vi "MainV2.vi"() -> ()   [LabVIEW 2010]
uses:
  <vilib>/Instr/_visa.llb/VISA Set IO Buffer Mask.ctl
  <vilib>/Instr/_visa.llb/VISA Flush IO Buffer Mask.ctl
  GlobalVar.vi
  <vilib>/Instr/_visa.llb/VISA Configure Serial Port (Instr).vi
panel:
  in  "Port Com":refnum<visa-resource-name>="COM7" caption="Nom de ressource VISA"
  in  "Bouton OK":bool
  in  "Data to send":dbl
  in  "Command type":u16(ring) items=["PRET"=53, "COEF_COURANT_2_INF"=36, "COEF_COURANT_2_CON"=164, "COEF_COURANT_1_INF"=35, "COEF_COURANT_1_CON"=163, "COEF_HYSTERISIS_SECURITE_INF"=34, "POURCENT_SECURITE_MOTEUR_INF"=33, "VITESSE_TROTTOIR_MAX_INF"=32, "DEMARRAGE_DELAI_EQUILIBRE_INF"=31, "DEMARRAGE_TOL_GUIDON_INF"=30, "DEMARRAGE_TOL_ANGLE_INF"=29, "LIMITE_DISTANCE_UTILISATEUR_INF"=28, "GUIDONMAX_INF"=27, "ACCELERATION_COEF_FILTRE_INF"=26, "COEF_KALMAN_INF"=25, "PRINC_DIR_INF"=24, "PRINC_PID_D_INF"=23, "PRINC_PID_K_INF"=22, "COEF_HYSTERISIS_SECURITE_CON"=162, "POURCENT_SECURITE_MOTEUR_CON"=161, "VITESSE_TROTTOIR_MAX_CON"=160, "DEMARRAGE_DELAI_EQUILIBRE_CON"=159, "DEMARRAGE_TOL_GUIDON_CON"=158, "DEMARRAGE_TOL_ANGLE_CON"=157, "LIMITE_DISTANCE_UTILISATEUR_CON"=156, "GUIDONMAX_CON"=155, "ACCELERATION_COEF_FILTRE_CON"=154, "COEF_KALMAN_CON"=153, "PRINC_DIR_CON"=152, "PRINC_PID_D_CON"=151, "PRINC_PID_K_CON"=150, "ENREGISTER_DEMARRAGE"=149, "CHARGER_DEMARRAGE"=148, "ENREGISTRER_ASSERVISSEMENT"=147, "CHARGER_ASSERVISSEMENT"=146, "ENREGISTRER_VITESSE"=145, "CHARGER_VITESSE"=144, "DEMANDE_COEFFICIENTS"=137, "VERBOSE_INF"=8, "VERBOSE_CON"=136, "ETAT"=1, "STOP"=131, "DEPART"=130, "TEST_COM"=129]
  out "LongToSend":u8
  out "TypeToSend":u8
  out "DataToSend":u8[](array[numeric])
  out "Frequency":dbl
  out "Enum":T1(ring)
  out "error":errorcluster
  out "error Connexion":errorcluster
  out "Stop main loop":bool
  in  "stop":bool
  in  "Tab Control":T2(tab)
  out "Reception":string
  in  "Comm_BaudRate":u32=9600 caption="Baud rate"
  in  "Comm_PortComm":refnum<visa-resource-name>="COM7" caption="Communication Port"
  in  "timeout (10sec)":u32=10000
  in  "Con_RefreshIntensity":bool caption="Bouton OK 12"
  in  "Con_RefreshRightTorque":bool caption="Bouton OK 12"
  out "Con_XYIntensity":cluster{"Y":dbl[], "Y":dbl[]}[](graph) caption="Intensity"
  out "Con_XYRightTorque":cluster{"Y":dbl[], "Y":dbl[]}[](graph) caption="Motor right Torque"
  in  "Con_RefreshLeftTorque":bool caption="Bouton OK 12"
  out "Con_XYLeftTorque":cluster{"Y":dbl[], "Y":dbl[]}[](graph) caption="Motor left Torque"
  out "Con_IntensityMax":bool caption="Max Intensity"
  out "Con_Intensity":string[][](array[string]) caption="Intensity (A)"
  out "Con_MotorRightTorque":string[][](array[string]) caption="Motor right Torque (N.m)"
  out "Con_MotorLeftTorque":string[][](array[string]) caption="Motor left Torque (N.m)"
  in  "Ana_RefreshBattery":bool caption="Bouton OK 12"
  out "Ana_XYBattery":cluster{"Y":dbl[], "Y":dbl[]}[](graph) caption="Motor left Torque"
  in  "Ana_RefreshHandlebar":bool caption="Bouton OK 12"
  out "Ana_XYHandlebar":cluster{"Y":dbl[], "Y":dbl[]}[](graph) caption="Motor left Torque"
  out "Ana_Battery":string[][](array[string]) caption="Battery"
  out "Ana_Handlebar":string[][](array[string]) caption="Handlebar"
  in  "Inc_RefreshAcceleration":bool caption="Bouton OK 12"
  out "Inc_XYAcceleration":cluster{"Y":dbl[], "Y":dbl[]}[](graph) caption="Motor left Torque"
  in  "Inc_RefreshVelocityRightMotor":bool caption="Bouton OK 12"
  out "Inc_XYVelocityRightMotor":cluster{"Y":dbl[], "Y":dbl[]}[](graph) caption="Motor left Torque"
  in  "Inc_RefreshVelocityLeftMotor":bool caption="Bouton OK 12"
  out "Inc_XYVelocityLeftMotor":cluster{"Y":dbl[], "Y":dbl[]}[](graph) caption="Motor left Torque"
  out "Inc_Acceleration":string[][](array[string]) caption="Acceleration"
  out "Inc_VelocityRightMotor":string[][](array[string]) caption="Velocity Right motor"
  out "Inc_VelocityLeftMotor":string[][](array[string]) caption="Velocity left motor"
  out "Other_AngularVelocity":string[][](array[string]) caption="Angular velocity"
  out "Other_AngleOUT":string[][](array[string]) caption="Angle Out of range"
  out "Other_SpeedSaturation":string[][](array[string]) caption="Speed saturation"
  out "Other_Distance":string[][](array[string]) caption="Distance"
  out "Other_Angle":string[][](array[string]) caption="Angle"
  in  "Analyse_Time":dbl caption="Time"
  in  "Analyse_Step":dbl caption="Step"
  in  "Analyse_LeftOrRight":bool caption="Booléen"
  out "Analyse_XYTorque":cluster{"Y":dbl[], "Y":dbl[]}[](graph) caption="Motor Torque command"
  out "Analyse_MotorTorque":string[][](array[string]) caption="Motor  Torque (N.m)"
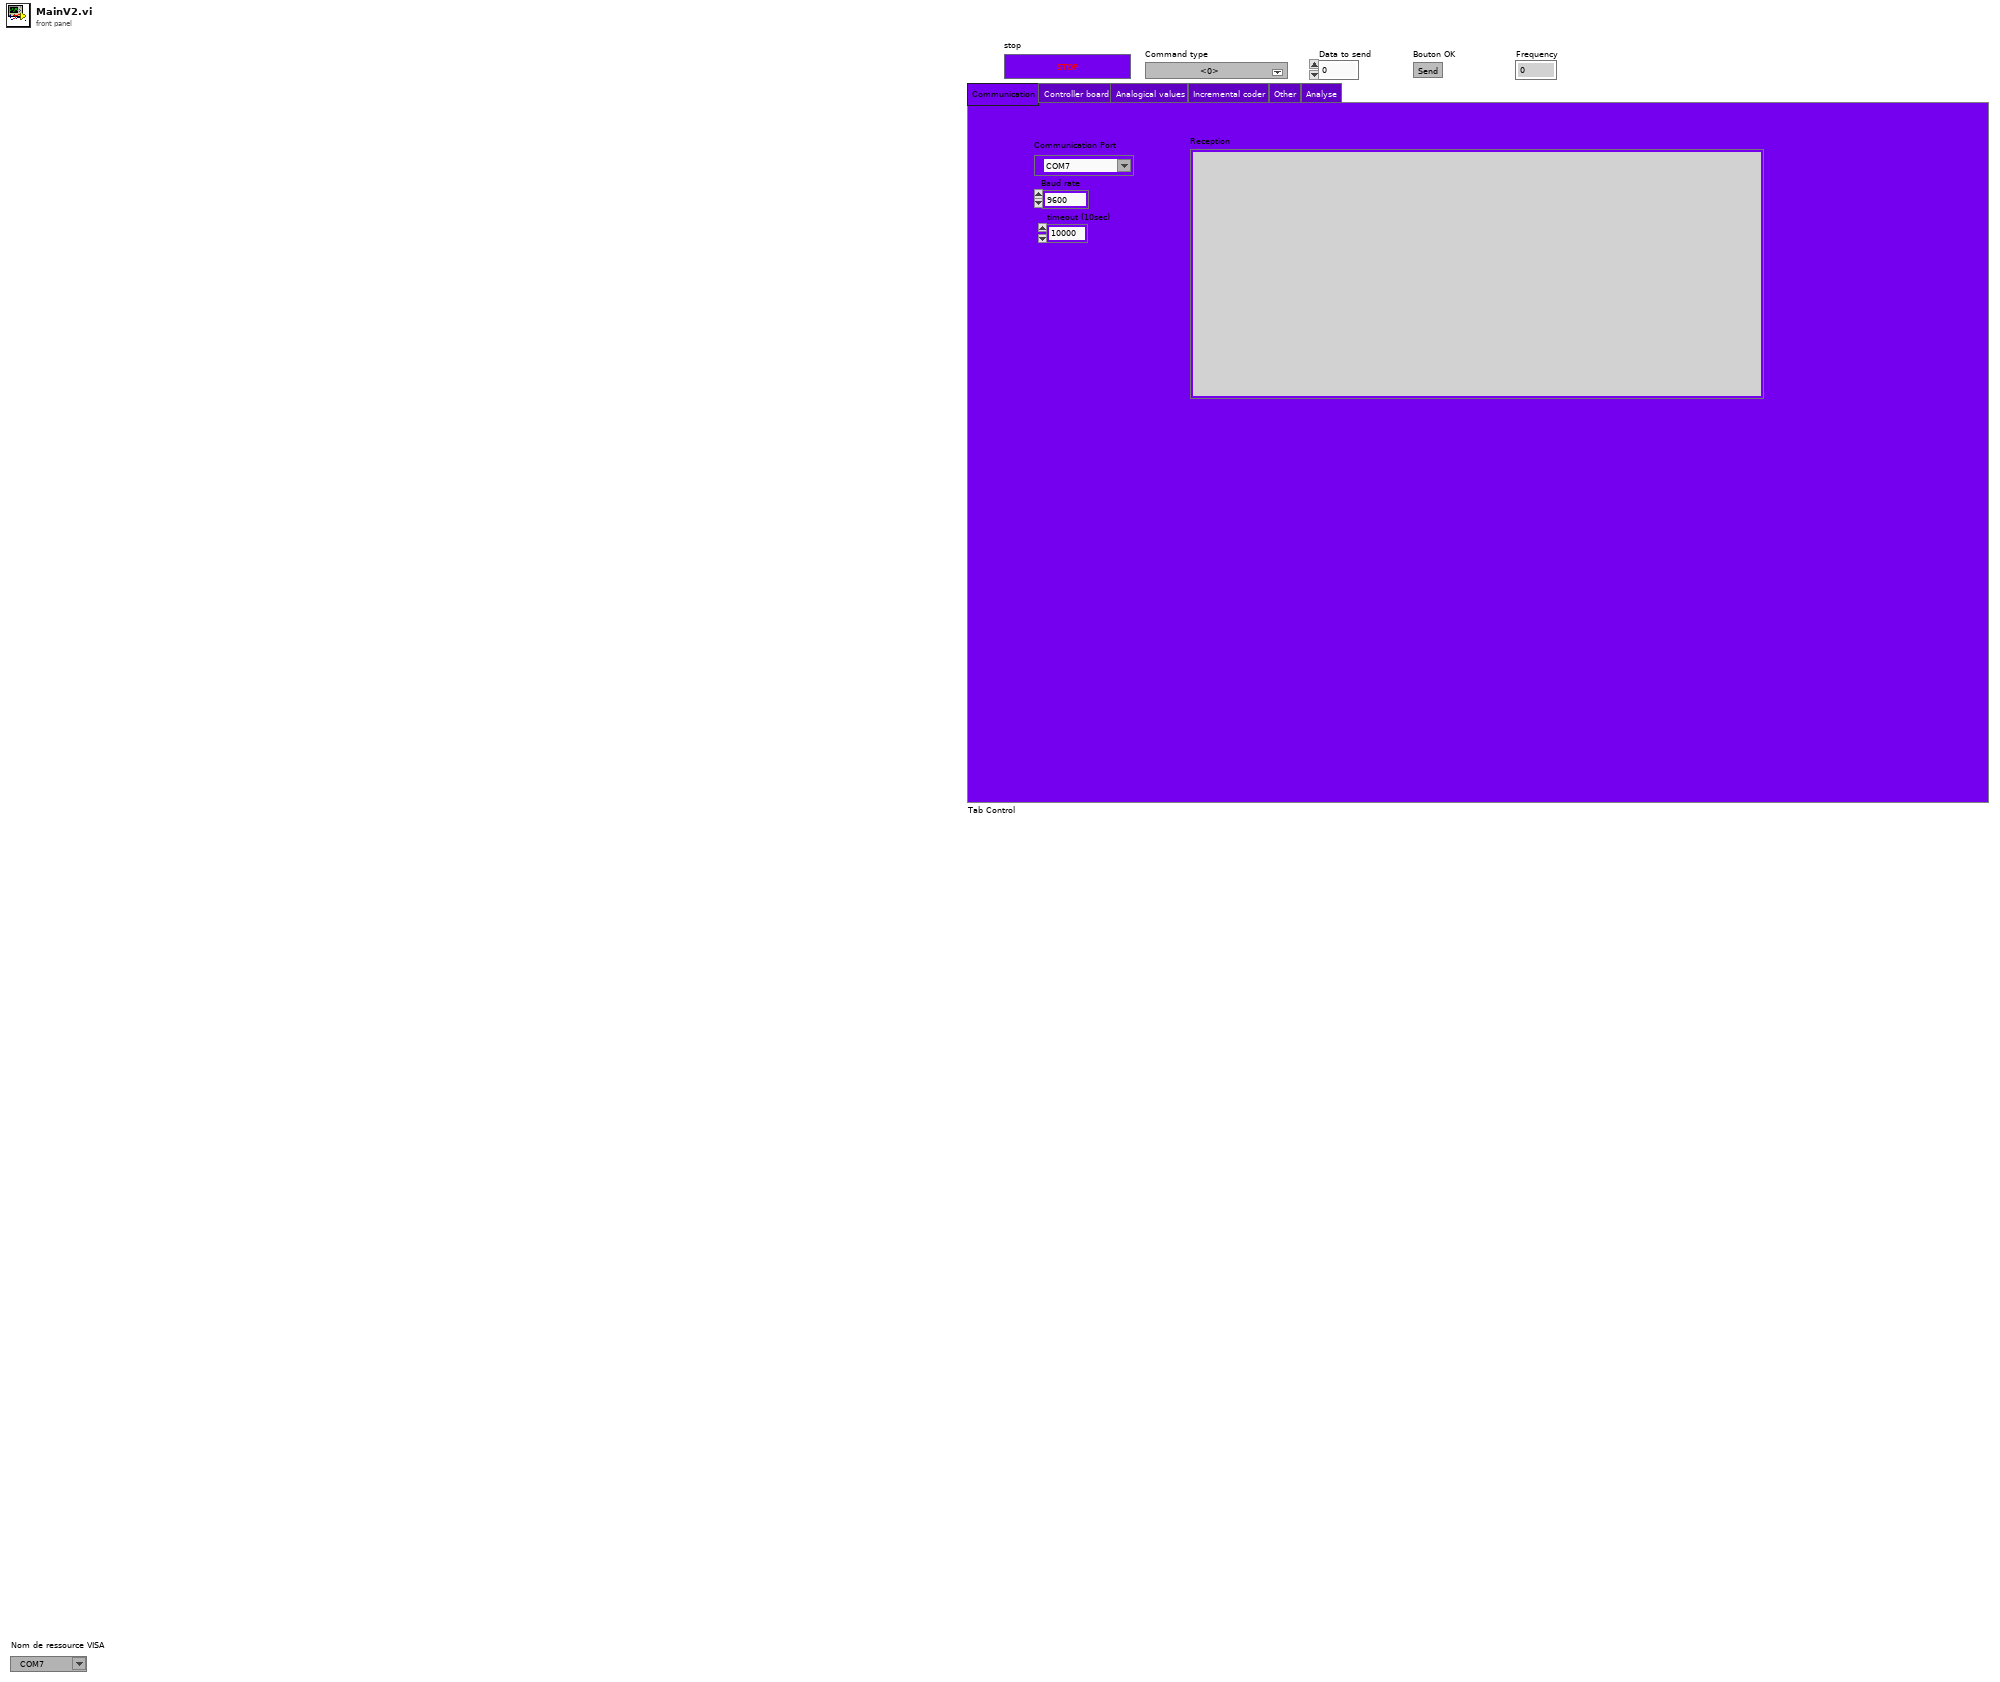
[diagram p1: front panel]
types:
  T1 = enum16{"Comm_TestConnection", "Con_RefreshLeftTorque", "Con_RefreshRightTorque", "Con_RefreshIntensity", "Ana_RefreshBattery", "Ana_RefreshHandlebar", "Inc_RefreshVelocityLeftMotor", "Inc_RefreshVelocityRightMotor", "Inc-RefreshAcceleration", "Spe_SendAnalysis", "Config_SendK", "Config_ReceiveK", "Config_SendD", "Config_ReceiveD", "Config_SendI", "Config_ReceiveI", "Config_SendCoefDir", "Config_ReceiveCoefDir", "Config_SendPID", "Config_SendCoefAcc", "Config_SendCoefKalman", "Config_ReceiveKalman", "Config_SendSTOP", "Config_SendRestart", "Config_SendCurrentState", "Config_SendReady", "Config_Sendvelocitysaturation", "Waiting"}
  T2 = enum32{"Communication", "Controller board", "Analogical values", "Incremental coder", "Other", "Analyse"}
  T3 = typedef "VISA Set IO Buffer Mask.ctl" = u16
  T4 = typedef "VISA Flush IO Buffer Mask.ctl" = u16
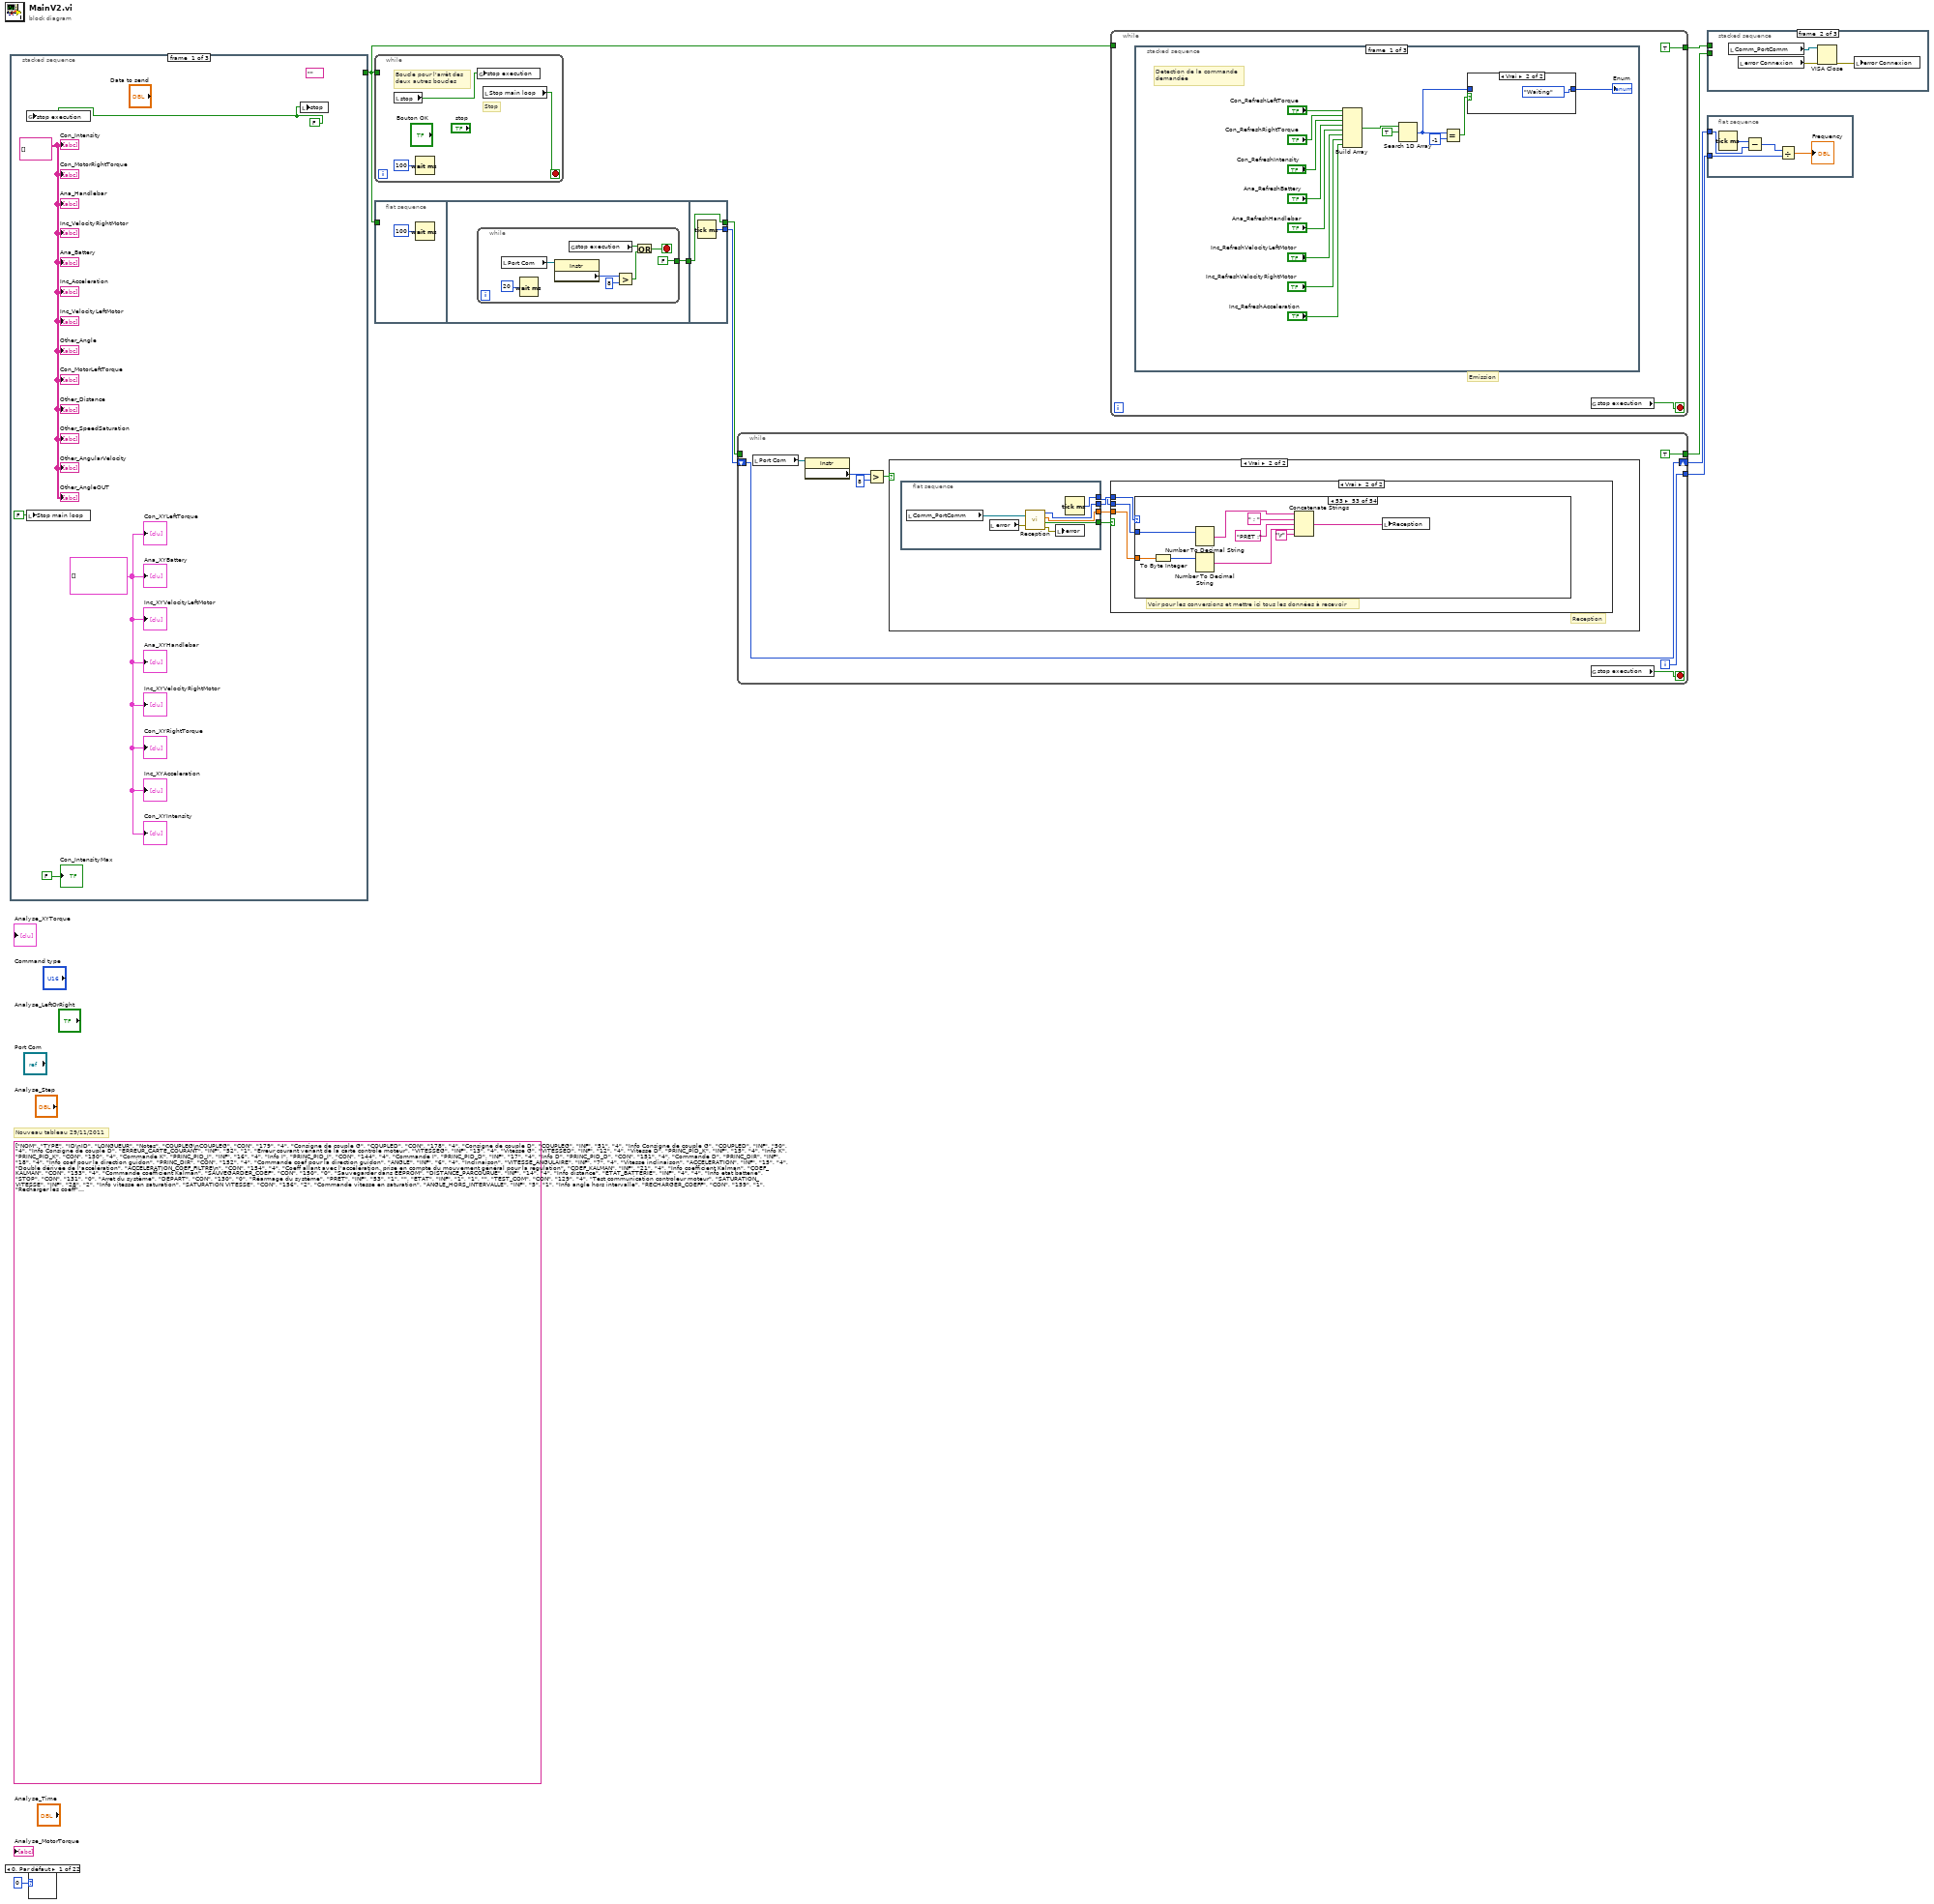
[diagram p0: block diagram]
diagram:
  (unwired) string[][] [["NOM", "TYPE", "ID\nID", "LONGUEUR", "Notes"], ["COUPLEG\nCOUPLEG", "CON", "179", "4", "Consigne de couple G"], ["COUPLED", "CON", "178", "4", "Consigne de couple D"], ["COUPLEG", "INF", "51", "4", "Info Consigne de couple G"], ["COUPLED", "INF", "50", "4", "Info Consigne de couple D"], ["ERREUR_CARTE_COURANT", "INF", "52", "1", "Erreur courant venant de la carte contrôle moteur"], ["VITESSEG", "INF", "13", "4", "Vitesse G"], ["VITESSED", "INF", "12", "4", "Vitesse D"], ["PRINC_PID_K", "INF", "15", "4", "Info K"], ["PRINC_PID_K", "CON", "150", "4", "Commande K"], ["PRINC_PID_I", "INF", "16", "4", "Info I"], ["PRINC_PID_I", "CON", "144", "4", "Commande I"], ["PRINC_PID_D", "INF", "17", "4", "Info D"], ["PRINC_PID_D", "CON", "151", "4", "Commande D"], ["PRINC_DIR", "INF", "18", "4", "Info coef pour la direction guidon"], ["PRINC_DIR", "CON", "152", "4", "Commande coef pour la direction guidon"], ["ANGLE", "INF", "6", "4", "Inclinaison"], ["VITESSE_ANGULAIRE", "INF", "7", "4", "Vitesse inclinaison"], ["ACCELERATION", "INF", "15", "4", "Double dérivée de l'accélération"], ["ACCELERATION_COEF_FILTRE\n", "CON", "154", "4", "Coeff allant avec l'accélération, prise en compte du mouvement général pour la régulation"], ["COEF_KALMAN", "INF", "21", "4", "Info coefficient Kalman"], ["COEF_KALMAN", "CON", "153", "4", "Commande coefficient Kalman"], ["SAUVEGARDER_COEF", "CON", "150", "0", "Sauvegarder dans EEPROM"], ["DISTANCE_PARCOURUE", "INF", "14", "4", "Info distance"], ["ETAT_BATTERIE", "INF", "4", "4", "Info etat batterie"], ["STOP", "CON", "131", "0", "Arret du système"], ["DEPART", "CON", "130", "0", "Réarmage du système"], ["PRET", "INF", "53", "1", ""], ["ETAT", "INF", "1", "1", ""], ["TEST_COM", "CON", "129", "4", "Test communication controleur moteur"], ["SATURATION_VITESSE", "INF", "28", "2", "Info vitesse en saturation"], ["SATURATION VITESSE", "CON", "156", "2", "Commande vitesse en saturation"], ["ANGLE_HORS_INTERVALLE", "INF", "5", "1", "Info angle hors intervalle"], ["RECHARGER_COEFF", "CON", "159", "1", "Recharger les coeff"], ["VERBOSE", "INF", "8", "2", ""], ["VERBOSE", "CON", "136", "2", ""], ["DEMANDE_COEFFICIENTS", "CON", "137", "1", ""], ["CHARGER_VITESSE", "CON", "144", "0", ""], ["ENREGISTRER_VITESSE", "CON", "145", "0", ""], ["CHARGER_ASSERVISSEMENT", "CON", "146", "0", ""], ["ENREGISTRER_ASSERVISSEMENT", "CON", "147", "0", ""], ["CHARGER_DEMARRAGE", "CON", "148", "0", ""], ["ENREGISTRER_DEMARRAGE", "CON", "149", "0", ""], ["GUIDONMAX", "INF", "27", "4", ""], ["LIMITE_DISTANCE_UTILISATEUR", "INF", "28", "4", ""], ["DEMARRAGE_TOL_ANGLE", "INF", "29", "4", ""], ["DEMARRAGE_TOL_GUIDON", "INF", "30", "4", ""], ["DEMARRAGE_DELAI_EQUILIBRE", "INF", "31", "4", ""], ["VITESSE_TROTTOIR_MAX", "INF", "32", "4", ""], ["POURCENT_SECURITE_MOTEUR", "INF", "33", "4", ""], ["COEF_HYSTERESIS_SECURITE", "INF", "34", "4", ""], ["COEF_COURANT_1", "CON", "163", "4", ""], ["COEF_COURANT_1", "INF", "35", "4", ""], ["COEF_COURANT_2", "CON", "164", "4", ""], ["COEF_COURANT_2", "INF", "36", "4", ""]]
  # "Nouveau tableau 29/11/2011"
  n1 = stacked-sequence {
    tunnel: [_ _ TRUE] -> w4
    frame #0 {
      (unwired) "" ("Spe_Liste")
      w13 = cluster{"Y":dbl[], "Y":dbl[]}[] [] ("Ana_XYHandlebar 3")
      w12 = string[][] [] ("Velocity motor left")
      w11 = FALSE ("Comm_LEDTest")
      n2 = global write "GlobalVar.vi" "stop execution"(w11) -> ()
      n3 = local write "Stop main loop"(FALSE ("Stop main loop")) -> ()
      n4 = local write "stop"(w11) -> ()
      "Con_IntensityMax" <- FALSE ("Con_IntensityMax")
      "Inc_Acceleration" <- w12
      "Other_Angle" <- w12
      "Other_SpeedSaturation" <- w12
      "Other_AngleOUT" <- w12
      "Other_Distance" <- w12
      "Ana_XYHandlebar" <- w13
      "Ana_XYBattery" <- w13
      "Inc_XYVelocityLeftMotor" <- w13
      "Inc_XYVelocityRightMotor" <- w13
      "Inc_XYAcceleration" <- w13
      "Con_MotorLeftTorque" <- w12
      "Con_MotorRightTorque" <- w12
      "Con_Intensity" <- w12
      "Inc_VelocityLeftMotor" <- w12
      "Inc_VelocityRightMotor" <- w12
      "Ana_Handlebar" <- w12
      "Ana_Battery" <- w12
      "Con_XYRightTorque" <- w13
      "Con_XYIntensity" <- w13
      "Con_XYLeftTorque" <- w13
      "Other_AngularVelocity" <- w12
    }
    frame #1 {
      w18 = T3 48 items=["Buffer d'entrées (E/S)"=16, "Buffer de sorties (E/S)"=32, "Buffer d'entrées et de sorties (E/S)"=48] ("Mask")
      w22 = T4 16 items=["Vider le buffer d'entrées"=16, "Écrire le buffer de sorties sur le périphérique"=32, "Vider le buffer d'entrées (Pas d'E/S)"=64, "Vider le buffer de sorties"=128] ("Mask")
      w25 = u16 0 items=["None"=0, "XON/XOFF"=1, "RTS/CTS"=2, "DTR/DSR"=4] ("flow control")
      w26 = u16 10 items=["1.0"=10, "1.5"=15, "2.0"=20] ("stop bits")
      w28 = u16 0 items=["None", "Odd", "Even", "Mark", "Space"] ("parity")
      # "Initial"
      n5 = local write "Tab Control"(T2."Communication" ("Tab Control")) -> ()
      n6 = call-poly "VISA Configure Serial Port"("VISA resource name"="Comm_PortComm", "timeout (10sec)"="timeout (10sec)", "baud rate (9600)"="Comm_BaudRate", "data bits (8)"=u16 8 ("data bits"), "parity (0:none)"=w28, "stop bits (10: 1 bit)"=w26, "flow control (0:none)"=w25) -> ("VISA resource name out"=w23:refnum<visa-resource-name>, "error out"=w20:errorcluster)  [unwired: 2 in, 5 out]
      "error Connexion" <- w20
      "error" <- w20
      n7 = VISA Set I/O Buffer Size(VISA resource name=w23, mask (16)=w18, size (4096)=u32 524288 ("taille (4096)"), error in (no error)=w20) -> (VISA resource name out=w21:refnum<visa-resource-name>, error out=w19:errorcluster)
      n8 = VISA Flush I/O Buffer(VISA resource name=w21, mask (16)=w22, error in (no error)=w19) -> ()  [unwired: 2 out]
      "Reception" <- "" ("Reception")
    }
    frame #2 {
      # "OK Initialisation"
    }
  }
  n9 = case shown="0, Par défaut" 0 {
    frame 0, Default {
    }
    frame 10 {
    }
    frame 11 {
    }
    frame 12 {
    }
    frame 13 {
    }
    frame 14 {
    }
    frame 15 {
    }
    frame 16 {
    }
    frame 17 {
    }
    frame 18 {
    }
    frame 19 {
    }
    frame 20 {
    }
    frame 21 {
    }
    frame 22 {
    }
    frame 23 {
    }
    frame 24 {
    }
    frame 25 {
    }
    frame 26 {
    }
    frame 27 {
    }
    frame 28 {
    }
    frame 29 {
    }
    frame 30 {
    }
  }
  n10 = while {
    tunnel: w4 -> [_]
    stop <- w33 stop-if-true
    # "Boucle pour l'arrêt des \ndeux autres boucles"
    # "Stop"
    n11 = local read "stop"() -> (w34:bool)
    n12 = Wait (ms)(milliseconds to wait=u32 100) -> ()  [unwired: 1 out]
    n13 = global write "GlobalVar.vi" "stop execution"(w34) -> ()
    n14 = local read "Stop main loop"() -> (w33:bool)
  }
  n15 = flat-sequence {
    tunnel: w4 -> [_]
    tunnel: [w36] -> w3
    tunnel: [w46] -> w5
    tunnel: w3 -> [w46]
    tunnel: [w45] -> w2
    frame #0 {
      n16 = Wait (ms)(milliseconds to wait=u32 100 ("attente (ms)")) -> ()  [unwired: 1 out]
    }
    frame #1 {
      n17 = while {
        tunnel: [FALSE] -> w36
        stop <- w37 stop-if-true
        n18 = local read "Port Com"() -> (w44:refnum<visa-resource-name>)
        n19 = Wait (ms)(milliseconds to wait=u32 20 ("attente (ms)")) -> ()  [unwired: 1 out]
        n20 = property class="Instr"(reference=w44) -> ("Serial Settings:Number of Bytes at Serial Port"=w43:u32)  [unwired: 1 in, 2 out]
        n21 = global read "GlobalVar.vi" "stop execution"() -> (w38:bool)
        n22 = Greater?(x=w43, y=u32 8) -> (0:w41:bool)
        n23 = Or(x=w38, y=w41) -> (x .or. y?=w37:bool)
      }
    }
    frame #2 {
      n24 = Tick Count (ms)() -> (millisecond timer value=w45:u32)
    }
  }
  n25 = while {
    tunnel: [TRUE] -> w9
    tunnel: [w52] -> w6
    tunnel: w5 -> [_]
    shift-right: [w51] -> w1
    shift-left: w2 -> [w51]
    i -> [w52]
    stop <- w53 stop-if-true
    n26 = local read "Port Com"() -> (w50:refnum<visa-resource-name>)
    n27 = property class="Instr"(reference=w50) -> ("Serial Settings:Number of Bytes at Serial Port"=w49:u32)  [unwired: 1 in, 2 out]
    n28 = Greater?(x=w49, y=u32 8) -> (0:w48:bool)
    n29 = case shown="Vrai" w48 {
      frame False {
      }
      frame True {
        # "Reception"
        n30 = flat-sequence {
          tunnel: [w63] -> w58
          tunnel: [w62] -> w57
          tunnel: [w61] -> w56
          tunnel: [w60] -> w55
          frame #0 {
            n31 = local read "Comm_PortComm"() -> (w65:refnum<visa-resource-name>)
            n32 = local read "error"() -> (w64:errorcluster)
            n33 = call "Reception.vi"("entrée d'erreur (pas d'erreur)"=w64, "Nom de ressource VISA"=w65) -> ("Sortie d'erreur"=w59:errorcluster, "Checksum OK?"=w63:bool, "Data"=w61:sgl, "ID byte"=w62:i32)
            n34 = local write "error"(w59) -> ()
            n35 = Tick Count (ms)() -> (millisecond timer value=w60:u32)
          }
        }
        n36 = case shown="Vrai" w58 {
          tunnel: w57 -> [_ w67]
          tunnel: w56 -> [_ w66]
          tunnel: w55 -> [_ w68]
          frame False {
          }
          frame True {
            # "Voir pour les conversions et mettre ici tous les données à recevoir"
            n37 = case shown="53" w67 {
              tunnel: w66 -> [_ w77 _ _ w79 w87 w96 w104 _ _ _ w112 w120 w128 w136 _ _ _ _ _ _ w144 w153 w162 w171 w181 w189 w198 w207 w216 w225 w234 w243 w252 w261 w270 _ _ _ _ _ _ _ _ _ _ _ _ _ w279 w286 w293 w301 w311]
              tunnel: w68 -> [_ w70 _ _ w78 w86 w95 w103 _ _ _ w111 w119 w127 w135 _ _ _ _ _ _ w143 w152 w161 w170 w180 w188 w197 w206 w215 w224 w233 w242 w251 w260 w269 _ _ _ _ _ _ _ _ _ _ _ _ _ w278 w285 w292 w302 w310]
              frame 0, Default {
              }
              frame 1 {
                n38 = To Byte Integer(number=w77) -> (8bit integer=w76:i8)
                n39 = Number To Decimal String(number=w70) -> (decimal integer string=w69:string)  [unwired: 1 in]
                n40 = Number To Decimal String(number=w76) -> (decimal integer string=w75:string)  [unwired: 1 in]
                n41 = Concatenate Strings(w69, " ; " ("chaîne"), "ETAT :" ("chaîne"), w75, "\r") -> (w72:string)
                n42 = local write "Reception"(w72) -> ()
              }
              frame 2 {
              }
              frame 3 {
              }
              frame 4 {
                n43 = Number To Decimal String(number=w78) -> (decimal integer string=w82:string)  [unwired: 1 in]
                n44 = Number To Exponential String(number=w79, precision (6)=i16 3 ("précision (6)")) -> (E-format string=w81:string)  [unwired: 2 in]
                n45 = local read "Ana_Battery"() -> (w80:string[][])
                n46 = Build Array(w81, w82) -> (w83:string[])
                n47 = Build Array (concatenate)(w80, w83) -> (w84:string[][])
                n48 = local write "Ana_Battery"(w84) -> ()
              }
              frame 5 {
                n49 = To Byte Integer(number=w87) -> (8bit integer=w94:i8)
                n50 = Number To Decimal String(number=w86) -> (decimal integer string=w88:string)  [unwired: 1 in]
                n51 = Number To Decimal String(number=w94) -> (decimal integer string=w93:string)  [unwired: 1 in]
                n52 = Concatenate Strings(w88, " ; " ("chaîne"), "ANGLE HORS INTERVALLE :" ("chaîne"), w93, "\r") -> (w90:string)
                n53 = local write "Reception"(w90) -> ()
              }
              frame 6 {
                n54 = Number To Decimal String(number=w95) -> (decimal integer string=w99:string)  [unwired: 1 in]
                n55 = Number To Exponential String(number=w96, precision (6)=i16 3 ("précision (6)")) -> (E-format string=w98:string)  [unwired: 2 in]
                n56 = local read "Other_Angle"() -> (w97:string[][])
                n57 = Build Array(w98, w99) -> (w100:string[])
                n58 = Build Array (concatenate)(w97, w100) -> (w101:string[][])
                n59 = local write "Other_Angle"(w101) -> ()
              }
              frame 7 {
                n60 = local read "Other_AngularVelocity"() -> (w105:string[][])
                n61 = Number To Decimal String(number=w103) -> (decimal integer string=w107:string)  [unwired: 1 in]
                n62 = Number To Exponential String(number=w104, precision (6)=i16 3 ("précision (6)")) -> (E-format string=w106:string)  [unwired: 2 in]
                n63 = Build Array(w106, w107) -> (w108:string[])
                n64 = Build Array (concatenate)(w105, w108) -> (w109:string[][])
                n65 = local write "Other_AngularVelocity"(w109) -> ()
              }
              frame 9 {
              }
              frame 10 {
              }
              frame 11 {
              }
              frame 12 {
                n66 = local read "Inc_VelocityRightMotor"() -> (w113:string[][])
                n67 = Number To Decimal String(number=w111) -> (decimal integer string=w115:string)  [unwired: 1 in]
                n68 = Number To Exponential String(number=w112, precision (6)=i16 3 ("précision (6)")) -> (E-format string=w114:string)  [unwired: 2 in]
                n69 = Build Array(w114, w115) -> (w116:string[])
                n70 = Build Array (concatenate)(w113, w116) -> (w117:string[][])
                n71 = local write "Inc_VelocityRightMotor"(w117) -> ()
              }
              frame 13 {
                n72 = local read "Inc_VelocityLeftMotor"() -> (w121:string[][])
                n73 = Number To Decimal String(number=w119) -> (decimal integer string=w123:string)  [unwired: 1 in]
                n74 = Number To Exponential String(number=w120, precision (6)=i16 3 ("précision (6)")) -> (E-format string=w122:string)  [unwired: 2 in]
                n75 = Build Array(w122, w123) -> (w124:string[])
                n76 = Build Array (concatenate)(w121, w124) -> (w125:string[][])
                n77 = local write "Inc_VelocityLeftMotor"(w125) -> ()
              }
              frame 14 {
                n78 = Number To Decimal String(number=w127) -> (decimal integer string=w131:string)  [unwired: 1 in]
                n79 = local read "Other_Distance"() -> (w129:string[][])
                n80 = Number To Exponential String(number=w128, precision (6)=i16 3 ("précision (6)")) -> (E-format string=w130:string)  [unwired: 2 in]
                n81 = Build Array(w130, w131) -> (w132:string[])
                n82 = Build Array (concatenate)(w129, w132) -> (w133:string[][])
                n83 = local write "Other_Distance"(w133) -> ()
              }
              frame 15 {
                n84 = local read "Inc_Acceleration"() -> (w137:string[][])
                n85 = Number To Decimal String(number=w135) -> (decimal integer string=w139:string)  [unwired: 1 in]
                n86 = Number To Exponential String(number=w136, precision (6)=i16 3 ("précision (6)")) -> (E-format string=w138:string)  [unwired: 2 in]
                n87 = Build Array(w138, w139) -> (w140:string[])
                n88 = Build Array (concatenate)(w137, w140) -> (w141:string[][])
                n89 = local write "Inc_Acceleration"(w141) -> ()
              }
              frame 16 {
              }
              frame 17 {
              }
              frame 18 {
              }
              frame 19 {
              }
              frame 20 {
              }
              frame 21 {
              }
              frame 22 {
                n90 = To Byte Integer(number=w144) -> (8bit integer=w151:i8)
                n91 = Number To Decimal String(number=w143) -> (decimal integer string=w145:string)  [unwired: 1 in]
                n92 = Number To Decimal String(number=w151) -> (decimal integer string=w150:string)  [unwired: 1 in]
                n93 = Concatenate Strings(w145, " ; " ("chaîne"), "PRINC_PID_K :" ("chaîne"), w150, "\r") -> (w147:string)
                n94 = local write "Reception"(w147) -> ()
              }
              frame 23 {
                n95 = To Byte Integer(number=w153) -> (8bit integer=w160:i8)
                n96 = Number To Decimal String(number=w152) -> (decimal integer string=w154:string)  [unwired: 1 in]
                n97 = Number To Decimal String(number=w160) -> (decimal integer string=w159:string)  [unwired: 1 in]
                n98 = Concatenate Strings(w154, " ; " ("chaîne"), "PRINC_PID_D :" ("chaîne"), w159, "\r") -> (w156:string)
                n99 = local write "Reception"(w156) -> ()
              }
              frame 24 {
                n100 = To Byte Integer(number=w162) -> (8bit integer=w169:i8)
                n101 = Number To Decimal String(number=w161) -> (decimal integer string=w163:string)  [unwired: 1 in]
                n102 = Number To Decimal String(number=w169) -> (decimal integer string=w168:string)  [unwired: 1 in]
                n103 = Concatenate Strings(w163, " ; " ("chaîne"), "PRINC_DIR :" ("chaîne"), w168, "\r") -> (w165:string)
                n104 = local write "Reception"(w165) -> ()
              }
              frame 25 {
                n105 = To Byte Integer(number=w171) -> (8bit integer=w178:i8)
                n106 = Number To Decimal String(number=w170) -> (decimal integer string=w172:string)  [unwired: 1 in]
                n107 = Number To Decimal String(number=w178) -> (decimal integer string=w177:string)  [unwired: 1 in]
                n108 = Concatenate Strings(w172, " ; " ("chaîne"), "COEF KALMAN :" ("chaîne"), w177, "\r") -> (w174:string)
                n109 = local write "Reception"(w174) -> ()
              }
              frame 26 {
                n110 = To Byte Integer(number=w181) -> (8bit integer=w187:i8)
                n111 = Number To Decimal String(number=w180) -> (decimal integer string=w179:string)  [unwired: 1 in]
                n112 = Number To Decimal String(number=w187) -> (decimal integer string=w186:string)  [unwired: 1 in]
                n113 = Concatenate Strings(w179, " ; " ("chaîne"), "ACCELERATION_COEF_FILTRE :" ("chaîne"), w186, "\r") -> (w183:string)
                n114 = local write "Reception"(w183) -> ()
              }
              frame 27 {
                n115 = To Byte Integer(number=w189) -> (8bit integer=w196:i8)
                n116 = Number To Decimal String(number=w188) -> (decimal integer string=w190:string)  [unwired: 1 in]
                n117 = Number To Decimal String(number=w196) -> (decimal integer string=w195:string)  [unwired: 1 in]
                n118 = Concatenate Strings(w190, " ; " ("chaîne"), "GUIDON_MAX :" ("chaîne"), w195, "\r") -> (w192:string)
                n119 = local write "Reception"(w192) -> ()
              }
              frame 28 {
                n120 = To Byte Integer(number=w198) -> (8bit integer=w205:i8)
                n121 = Number To Decimal String(number=w197) -> (decimal integer string=w199:string)  [unwired: 1 in]
                n122 = Number To Decimal String(number=w205) -> (decimal integer string=w204:string)  [unwired: 1 in]
                n123 = Concatenate Strings(w199, " ; " ("chaîne"), "LIMITE_DISTANCE_UTILISATEUR :" ("chaîne"), w204, "\r") -> (w201:string)
                n124 = local write "Reception"(w201) -> ()
              }
              frame 29 {
                n125 = To Byte Integer(number=w207) -> (8bit integer=w214:i8)
                n126 = Number To Decimal String(number=w206) -> (decimal integer string=w208:string)  [unwired: 1 in]
                n127 = Number To Decimal String(number=w214) -> (decimal integer string=w213:string)  [unwired: 1 in]
                n128 = Concatenate Strings(w208, " ; " ("chaîne"), "DEMARRAGE_TOL_ANGLE :" ("chaîne"), w213, "\r") -> (w210:string)
                n129 = local write "Reception"(w210) -> ()
              }
              frame 30 {
                n130 = To Byte Integer(number=w216) -> (8bit integer=w223:i8)
                n131 = Number To Decimal String(number=w215) -> (decimal integer string=w217:string)  [unwired: 1 in]
                n132 = Number To Decimal String(number=w223) -> (decimal integer string=w222:string)  [unwired: 1 in]
                n133 = Concatenate Strings(w217, " ; " ("chaîne"), "DEMARRAGE_TOL_GUIDON :" ("chaîne"), w222, "\r") -> (w219:string)
                n134 = local write "Reception"(w219) -> ()
              }
              frame 31 {
                n135 = To Byte Integer(number=w225) -> (8bit integer=w232:i8)
                n136 = Number To Decimal String(number=w224) -> (decimal integer string=w226:string)  [unwired: 1 in]
                n137 = Number To Decimal String(number=w232) -> (decimal integer string=w231:string)  [unwired: 1 in]
                n138 = Concatenate Strings(w226, " ; " ("chaîne"), "DEMARRAGE_DELAI_EQUILIBRE :" ("chaîne"), w231, "\r") -> (w228:string)
                n139 = local write "Reception"(w228) -> ()
              }
              frame 32 {
                n140 = To Byte Integer(number=w234) -> (8bit integer=w241:i8)
                n141 = Number To Decimal String(number=w233) -> (decimal integer string=w235:string)  [unwired: 1 in]
                n142 = Number To Decimal String(number=w241) -> (decimal integer string=w240:string)  [unwired: 1 in]
                n143 = Concatenate Strings(w235, " ; " ("chaîne"), "VITESSE_TROTTOIR_MAX :" ("chaîne"), w240, "\r") -> (w237:string)
                n144 = local write "Reception"(w237) -> ()
              }
              frame 33 {
                n145 = To Byte Integer(number=w243) -> (8bit integer=w250:i8)
                n146 = Number To Decimal String(number=w242) -> (decimal integer string=w244:string)  [unwired: 1 in]
                n147 = Number To Decimal String(number=w250) -> (decimal integer string=w249:string)  [unwired: 1 in]
                n148 = Concatenate Strings(w244, " ; " ("chaîne"), "POURCENT_SECURITE_MOTEUR :" ("chaîne"), w249, "\r") -> (w246:string)
                n149 = local write "Reception"(w246) -> ()
              }
              frame 34 {
                n150 = To Byte Integer(number=w252) -> (8bit integer=w259:i8)
                n151 = Number To Decimal String(number=w251) -> (decimal integer string=w253:string)  [unwired: 1 in]
                n152 = Number To Decimal String(number=w259) -> (decimal integer string=w258:string)  [unwired: 1 in]
                n153 = Concatenate Strings(w253, " ; " ("chaîne"), "COEF_HYSTERISIS :" ("chaîne"), w258, "\r") -> (w255:string)
                n154 = local write "Reception"(w255) -> ()
              }
              frame 35 {
                n155 = To Byte Integer(number=w261) -> (8bit integer=w268:i8)
                n156 = Number To Decimal String(number=w260) -> (decimal integer string=w262:string)  [unwired: 1 in]
                n157 = Number To Decimal String(number=w268) -> (decimal integer string=w267:string)  [unwired: 1 in]
                n158 = Concatenate Strings(w262, " ; " ("chaîne"), "COEF_COURANT_1 :" ("chaîne"), w267, "\r") -> (w264:string)
                n159 = local write "Reception"(w264) -> ()
              }
              frame 36 {
                n160 = To Byte Integer(number=w270) -> (8bit integer=w277:i8)
                n161 = Number To Decimal String(number=w269) -> (decimal integer string=w271:string)  [unwired: 1 in]
                n162 = Number To Decimal String(number=w277) -> (decimal integer string=w276:string)  [unwired: 1 in]
                n163 = Concatenate Strings(w271, " ; " ("chaîne"), "COEF_COURANT_2 :" ("chaîne"), w276, "\r") -> (w273:string)
                n164 = local write "Reception"(w273) -> ()
              }
              frame 37 {
              }
              frame 38 {
              }
              frame 39 {
              }
              frame 40 {
              }
              frame 41 {
              }
              frame 42 {
              }
              frame 43 {
              }
              frame 44 {
              }
              frame 45 {
              }
              frame 46 {
              }
              frame 47 {
              }
              frame 48 {
              }
              frame 49 {
              }
              frame 50 {
                n165 = Number To Decimal String(number=w278) -> (decimal integer string=w282:string)  [unwired: 1 in]
                n166 = Number To Decimal String(number=w279) -> (decimal integer string=w281:string)  [unwired: 1 in]
                n167 = Build Array(w281, w282) -> (w283:string[])
                n168 = local read "Con_MotorRightTorque"() -> (w280:string[][])
                n169 = Build Array (concatenate)(w280, w283) -> (w284:string[][])
                n170 = local write "Con_MotorRightTorque"(w284) -> ()
              }
              frame 51 {
                n171 = Number To Decimal String(number=w285) -> (decimal integer string=w289:string)  [unwired: 1 in]
                n172 = Number To Decimal String(number=w286) -> (decimal integer string=w288:string)  [unwired: 1 in]
                n173 = Build Array(w288, w289) -> (w290:string[])
                n174 = local read "Con_MotorLeftTorque"() -> (w287:string[][])
                n175 = Build Array (concatenate)(w287, w290) -> (w291:string[][])
                n176 = local write "Con_MotorLeftTorque"(w291) -> ()
              }
              frame 52 {
                n177 = To Byte Integer(number=w293) -> (8bit integer=w300:i8)
                n178 = Number To Decimal String(number=w292) -> (decimal integer string=w294:string)  [unwired: 1 in]
                n179 = Number To Decimal String(number=w300) -> (decimal integer string=w299:string)  [unwired: 1 in]
                n180 = Concatenate Strings(w294, " ; " ("chaîne"), "ERREUR CARTE COURANT :" ("chaîne"), w299, "\r") -> (w296:string)
                n181 = local write "Reception"(w296) -> ()
              }
              frame 53 {
                n182 = To Byte Integer(number=w301) -> (8bit integer=w309:i8)
                n183 = Number To Decimal String(number=w302) -> (decimal integer string=w303:string)  [unwired: 1 in]
                n184 = Number To Decimal String(number=w309) -> (decimal integer string=w308:string)  [unwired: 1 in]
                n185 = Concatenate Strings(w303, " ; " ("chaîne"), "PRET :" ("chaîne"), w308, "\r") -> (w305:string)
                n186 = local write "Reception"(w305) -> ()
              }
              frame 8 {
                n187 = To Byte Integer(number=w311) -> (8bit integer=w318:i8)
                n188 = Number To Decimal String(number=w310) -> (decimal integer string=w312:string)  [unwired: 1 in]
                n189 = Number To Decimal String(number=w318) -> (decimal integer string=w317:string)  [unwired: 1 in]
                n190 = Concatenate Strings(w312, " ; " ("chaîne"), "VERBOSE :" ("chaîne"), w317, "\r") -> (w314:string)
                n191 = local write "Reception"(w314) -> ()
              }
            }
          }
        }
      }
    }
    n192 = global read "GlobalVar.vi" "stop execution"() -> (w53:bool)
  }
  n193 = while {
    tunnel: w4 -> [_]
    tunnel: [TRUE] -> w8
    stop <- w319 stop-if-true
    # "Emission"
    n194 = stacked-sequence {
      frame #0 {
        # "Detection de la commande\ndemandée"
        n195 = Build Array("Con_RefreshLeftTorque", "Con_RefreshRightTorque", "Con_RefreshIntensity", "Ana_RefreshBattery", "Ana_RefreshHandlebar", "Inc_RefreshVelocityLeftMotor", "Inc_RefreshVelocityRightMotor", "Inc_RefreshAcceleration") -> (w334:bool[])
        n196 = Search 1D Array(1D array=w334, element=TRUE) -> (index of element=w330:i32)  [unwired: 1 in]
        n197 = Equal?(x=w330, y=-1) -> (x = y?=w332:bool)
        n198 = case shown="Vrai" w332 {
          tunnel: [w335 T1."Waiting" ("Enum 2")] -> w331
          tunnel: w330 -> [w335 _]
          frame False {
          }
          frame True {
          }
        }
        "Enum" <- w331
      }
      frame #1 {
        # "Traitement de la commande,\nboucles pour des mesures avec création \nde la trame série,\nautre pour la configuration"
        n199 = local read "Enum"() -> (w337:T1)
        n200 = case shown="\"Config_SendK\"" w337 {
          frame "Comm_TestConnection" {
            n201 = One Button Dialog(message="Not available.") -> ()  [unwired: 1 in, 1 out]
          }
          frame "Con_RefreshRightTorque" {
            n202 = local read "Con_MotorRightTorque"() -> (w340:string[][])
            n203 = call "TableToXYGraph.vi"("Input Table"=w340) -> ("XY Graph"=w339:cluster{"Y":dbl[], "Y":dbl[]}[])
            n204 = local write "Con_XYRightTorque"(w339) -> ()
          }
          frame "Con_RefreshIntensity" {
            n205 = local read "Con_Intensity"() -> (w342:string[][])
            n206 = call "TableToXYGraph.vi"("Input Table"=w342) -> ("XY Graph"=w341:cluster{"Y":dbl[], "Y":dbl[]}[])
            n207 = local write "Con_XYIntensity"(w341) -> ()
          }
          frame "Ana_RefreshBattery" {
            n208 = local read "Ana_Battery"() -> (w344:string[][])
            n209 = call "TableToXYGraph.vi"("Input Table"=w344) -> ("XY Graph"=w343:cluster{"Y":dbl[], "Y":dbl[]}[])
            n210 = local write "Ana_XYBattery"(w343) -> ()
          }
          frame "Ana_RefreshHandlebar" {
            n211 = local read "Ana_Handlebar"() -> (w346:string[][])
            n212 = call "TableToXYGraph.vi"("Input Table"=w346) -> ("XY Graph"=w345:cluster{"Y":dbl[], "Y":dbl[]}[])
            n213 = local write "Ana_XYHandlebar"(w345) -> ()
          }
          frame "Inc_RefreshVelocityLeftMotor" {
            n214 = local read "Inc_VelocityLeftMotor"() -> (w348:string[][])
            n215 = call "TableToXYGraph.vi"("Input Table"=w348) -> ("XY Graph"=w347:cluster{"Y":dbl[], "Y":dbl[]}[])
            n216 = local write "Inc_XYVelocityLeftMotor"(w347) -> ()
          }
          frame "Inc_RefreshVelocityRightMotor" {
            n217 = local read "Inc_VelocityRightMotor"() -> (w350:string[][])
            n218 = call "TableToXYGraph.vi"("Input Table"=w350) -> ("XY Graph"=w349:cluster{"Y":dbl[], "Y":dbl[]}[])
            n219 = local write "Inc_XYVelocityRightMotor"(w349) -> ()
          }
          frame "Inc-RefreshAcceleration" {
            n220 = local read "Inc_Acceleration"() -> (w352:string[][])
            n221 = call "TableToXYGraph.vi"("Input Table"=w352) -> ("XY Graph"=w351:cluster{"Y":dbl[], "Y":dbl[]}[])
            n222 = local write "Inc_XYAcceleration"(w351) -> ()
          }
          frame "Spe_SendAnalysis" {
            n223 = One Button Dialog(message="Not available.") -> ()  [unwired: 1 in, 1 out]
          }
          frame "Config_SendK" {
            w358 = u8[] []  # type U8
            n224 = local write "LongToSend"(u8 4 ("LongToSend")) -> ()
            n225 = local write "TypeToSend"(u8 143 ("TypeToSend")) -> ()
            n226 = Type Cast(type=w358, x=ext 0.0) -> (*(type *) &x=w357:u8[])
            n227 = local write "DataToSend"(w357) -> ()
          }
          frame "Config_ReceiveK" {
            n228 = One Button Dialog(message="Not available.") -> ()  [unwired: 1 in, 1 out]
          }
          frame "Config_SendD" {
            n229 = One Button Dialog(message="Not available.") -> ()  [unwired: 1 in, 1 out]
          }
          frame "Config_ReceiveD" {
            n230 = One Button Dialog(message="Not available.") -> ()  [unwired: 1 in, 1 out]
          }
          frame "Config_SendI" {
            n231 = One Button Dialog(message="Not available.") -> ()  [unwired: 1 in, 1 out]
          }
          frame "Config_ReceiveI" {
            n232 = One Button Dialog(message="Not available.") -> ()  [unwired: 1 in, 1 out]
          }
          frame "Config_SendCoefDir" {
            n233 = One Button Dialog(message="Not available.") -> ()  [unwired: 1 in, 1 out]
          }
          frame "Config_ReceiveCoefDir" {
            n234 = One Button Dialog(message="Not available.") -> ()  [unwired: 1 in, 1 out]
          }
          frame "Config_SendPID" {
            n235 = One Button Dialog(message="Not available.") -> ()  [unwired: 1 in, 1 out]
          }
          frame "Config_SendCoefAcc" {
            n236 = One Button Dialog(message="Not available.") -> ()  [unwired: 1 in, 1 out]
          }
          frame "Config_SendCoefKalman" {
            n237 = One Button Dialog(message="Not available.") -> ()  [unwired: 1 in, 1 out]
          }
          frame "Config_ReceiveKalman" {
            n238 = One Button Dialog(message="Not available.") -> ()  [unwired: 1 in, 1 out]
          }
          frame "Config_SendSTOP" {
            n239 = One Button Dialog(message="Not available.") -> ()  [unwired: 1 in, 1 out]
          }
          frame "Config_SendRestart" {
            n240 = One Button Dialog(message="Not available.") -> ()  [unwired: 1 in, 1 out]
          }
          frame "Config_SendCurrentState" {
            n241 = One Button Dialog(message="Not available.") -> ()  [unwired: 1 in, 1 out]
          }
          frame "Config_SendReady" {
            n242 = One Button Dialog(message="Not available.") -> ()  [unwired: 1 in, 1 out]
          }
          frame "Config_Sendvelocitysaturation" {
            n243 = One Button Dialog(message="Not available.") -> ()  [unwired: 1 in, 1 out]
          }
          frame "Waiting", Default {
          }
          frame "Con_RefreshLeftTorque" {
            n244 = local read "Con_MotorLeftTorque"() -> (w376:string[][])
            n245 = call "TableToXYGraph.vi"("Input Table"=w376) -> ("XY Graph"=w375:cluster{"Y":dbl[], "Y":dbl[]}[])
            n246 = local write "Con_XYLeftTorque"(w375) -> ()
          }
        }
      }
      frame #2 {
        # "Envoyer la trame"
        n247 = local read "Comm_PortComm"() -> (w377:refnum<visa-resource-name>)
        n248 = local read "TypeToSend"() -> (w379:u8)
        n249 = local read "DataToSend"() -> (w378:u8[])
        n250 = local read "error"() -> (w380:errorcluster)
        n251 = call "Send.vi"("entrée d'erreur (pas d'erreur)"=w380, "tableau d'octets non signés"=w378, "Type"=w379, "Nom de ressource VISA"=w377) -> ("sortie d'erreur"=w381:errorcluster)
        n252 = local write "error"(w381) -> ()
      }
    }
    n253 = global read "GlobalVar.vi" "stop execution"() -> (w319:bool)
  }
  n254 = stacked-sequence {
    tunnel: w9 -> [_ _ _]
    tunnel: w8 -> [w382 _ _]
    frame #0 {
      # "Finalisation"
      "Stop main loop" <- w382
    }
    frame #1 {
      n255 = local read "Comm_PortComm"() -> (w385:refnum<visa-resource-name>)
      n256 = local read "error Connexion"() -> (w384:errorcluster)
      n257 = VISA Close(VISA resource name=w385, error in (no error)=w384) -> (error out=w383:errorcluster)
      n258 = local write "error Connexion"(w383) -> ()
    }
    frame #2 {
      n259 = local read "error Connexion"() -> (w388:errorcluster)
      n260 = local read "error"() -> (w387:errorcluster)
      n261 = Merge Errors(w387, w388) -> (w386:errorcluster)
      n262 = call <vilib>:"Simple Error Handler.vi"("error in (no error)"=w386) -> ()  [unwired: 4 in, 5 out]
    }
  }
  n263 = flat-sequence {
    tunnel: w6 -> [w391]
    tunnel: w1 -> [w389]
    frame #0 {
      n264 = Tick Count (ms)() -> (millisecond timer value=w393:u32)
      n265 = Subtract(x=w393, y=w389) -> (x-y=w392:u32)
      n266 = Divide(x=w392, y=w391) -> (x/y=→"Frequency":dbl)
    }
  }
